vi "DO_WF_NumberSamples.vi"(8 "error in":errorcluster, 10 "Action":enum16{"Init", "Write", "Read"}(ring), 11 "DO_WF_NumberOfSamples":u32=1000) -> (0 "error out":errorcluster, 3 "DO_WF_NumberOfSamples":u32=1000)   [LabVIEW 2025]
doc: "Functional Global Variable:\n- Write the value into the memory \nor\n- Read the value from the memory"
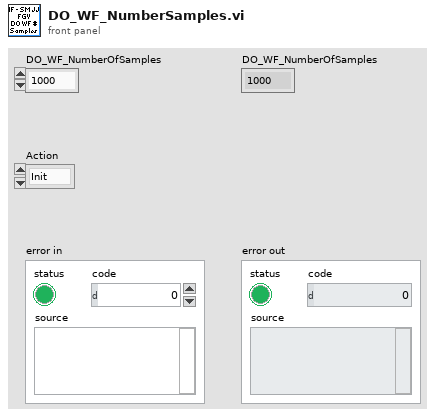
[diagram p1: front panel]
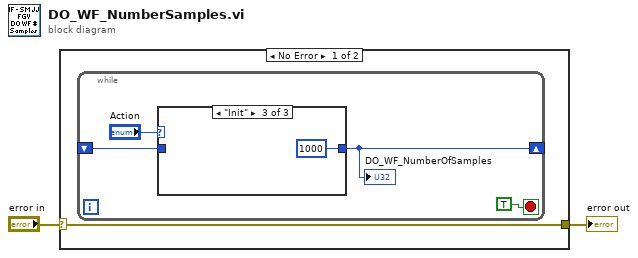
[diagram p0: block diagram]
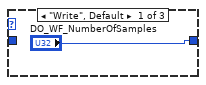
[diagram p2: hidden frame]
diagram:
  n1 = case shown="No Error" "error in" {
    selector: "error in" -> [w3 w11]
    tunnel: [w3 w11] -> w1
    frame No Error {
      n2 = while {
        shift-right: [w4] -> _
        shift-left: _ -> [w5]
        stop <- TRUE stop-if-true
        n3 = case shown="\"Init\"" "Action" {
          tunnel: w5 -> [_ w9 _]
          tunnel: ["DO_WF_NumberOfSamples" w9 u32 1000 ("DO_WF_NumberOfSamples")] -> w4
          frame "Write", Default {
          }
          frame "Read" {
          }
          frame "Init" {
          }
        }
        "DO_WF_NumberOfSamples" <- w4
      }
    }
    frame Error {
    }
  }
  "error out" <- w1
